vi "Send Request Message.vi"(4 "reply-topic":string, 6 "id":string, 7 "Qualified Name":string, 8 "error in":errorcluster, 9 "<JSON>params":string="{}", 10 "method":string, 11 "Actor Class":T1) -> (0 "error out":errorcluster, 1 "id out":string, 2 "method dup":string)   [LabVIEW 2019]
uses:
  Actor Private Data.ctl
  <vilib>/LabVIEW Open Source Project/MQTT Client/Client class/Client.lvclass
  Actor Private Events -- cluster.ctl
  Payload -- cluster.ctl
  Request -- cluster.ctl
  93570760-5aeb-4778-8a40-a1296721cb8c.vi
  <vilib>/JDP Science/JSONtext/Variant to JSON Text.vi
  <vilib>/JDP Science/JSONtext/LVClass Serializer/JSONtext LVClass Serializer.lvclass
  <vilib>/LabVIEW Open Source Project/Unicity/RandomStringGenerator/RandomStringGenerator.lvclass
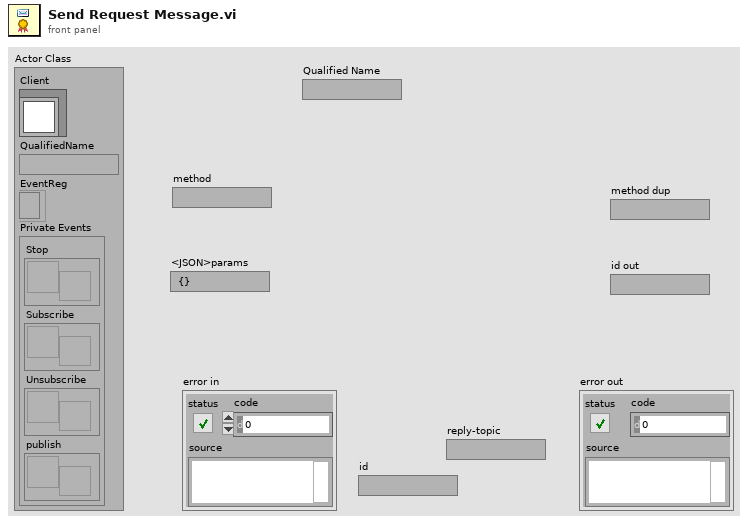
[diagram p1: front panel]
types:
  T1 = typedef "Actor Private Data.ctl" = cluster{"Client":refnum<class "Client.lvclass">, "QualifiedName":string, "EventReg":refnum<event-registration>, "Private Events":T2}
  T2 = typedef "Actor Private Events -- cluster.ctl" = cluster{"Stop":refnum<user-event>, "Subscribe":refnum<user-event>, "Unsubscribe":refnum<user-event>, "publish":refnum<user-event>}
  T3 = typedef "Request -- cluster.ctl" = cluster{"method":string, "<JSON>params":string, "id":string, "reply-topic":string}
  T4 = typedef "Payload -- cluster.ctl" = cluster{"topic":string, "Payload":u8[]}
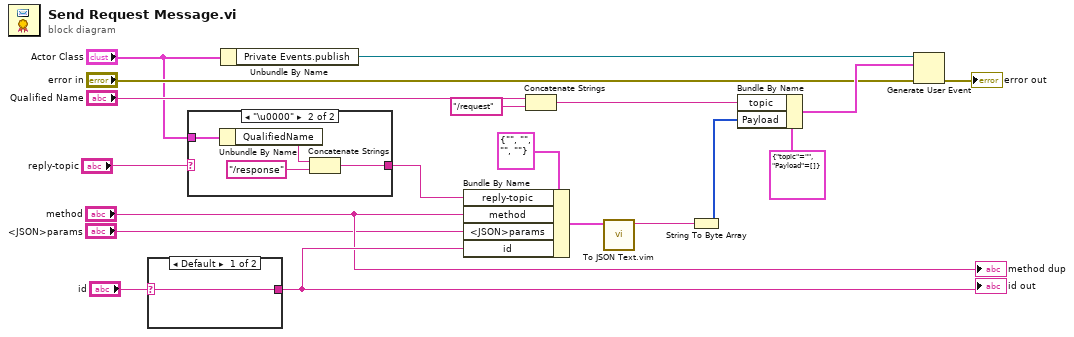
[diagram p0: block diagram]
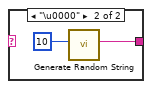
[diagram p3: hidden frame]
diagram:
  n1 = case shown="Default" "id" {
    selector: "id" -> [w20 _]
    tunnel: [w20 w21] -> w5
    frame Default {
    }
    frame "\u0000" {
      n2 = call <vilib>:"Generate Random String.vi"("String Length (32)"=u32 10) -> ("Random String"=w21:string)  [unwired: 10 in]
    }
  }
  "id out" <- w5
  n3 = case shown="\"\"" "reply-topic" {
    selector: "reply-topic" -> [w23 _]
    tunnel: "Actor Class" -> [_ w27]
    tunnel: [w23 w24] -> w6
    frame Default {
    }
    frame "\u0000" {
      n4 = Unbundle By Name(w27) -> ("QualifiedName"=w25:string)
      n5 = Concatenate Strings(w25, "/response" ("string")) -> (w24:string)
    }
  }
  n6 = Unbundle By Name("Actor Class") -> ("Private Events.publish"=w15:refnum<user-event>)
  n7 = Bundle By Name(cluster=T3 {"method"="", "<JSON>params"="", "id"="", "reply-topic"=""} ("request"), "reply-topic"=w6, "method"="method", "<JSON>params"="<JSON>params", "id"=w5) -> (w9:T3)
  n8 = Concatenate Strings("Qualified Name", "/request" ("string")) -> (w12:string)
  n9 = call "To JSON Text.vim"("Anything"=w9) -> ("<JSON>"=w8:string)  [unwired: 9 in, 1 out]
  n10 = String To Byte Array(string=w8) -> (unsigned byte array=w10:u8[])
  n11 = Bundle By Name(cluster=T4 {"topic"="", "Payload"=[]} ("publish"), "topic"=w12, "Payload"=w10) -> (w18:T4)
  n12 = Generate User Event(user event=w15, event data cluster=w18, error in="error in") -> (error out=→"error out":errorcluster)  [unwired: 1 in, 1 out]
  "method dup" <- "method"
